vi "Ctor.vi"(8 "error in (no error)":errorcluster) -> (0 "error out":errorcluster, 3 "AST out":refnum<class "AST.lvclass">)   [LabVIEW 2020, in "PicoG-ParserLexer.lvlib" / "AST.lvclass"]
uses:
  AST.lvclass
  Symbol Map/Symbol Map.lvclass
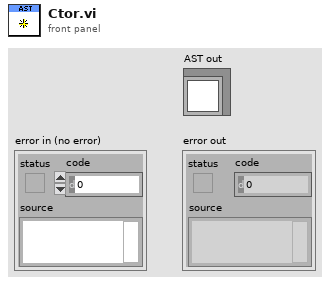
[diagram p1: front panel]
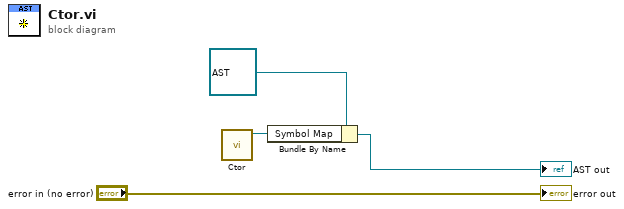
[diagram p0: block diagram]
diagram:
  n1 = call "Ctor.vi"() -> ("Symbol Map out"=w1:refnum<class "Symbol Map.lvclass">)  [unwired: 10 in, 1 out]
  n2 = Bundle By Name(cluster=refnum<class "AST.lvclass"> refnum ("AST out"), "Symbol Map"=w1) -> (→"AST out":refnum<class "AST.lvclass">)
  "error out" <- "error in (no error)"
